vi "Ver 1.7.vi"() -> ()   [LabVIEW 2015]
uses:
  <instrlib>/Keithley 622x LV 2009/Configure/Source/Typedefs/KE622x -- Current Range.ctl
  <instrlib>/Keithley 622x LV 2009/Configure/Source/Typedefs/KE622x -- Current Ranges.ctl
  <instrlib>/Keithley 622x LV 2009/Typedefs/KE622x -- On Off Control.ctl
  <instrlib>/Keithley 622x LV 2009/Configure/Source/Typedefs/KE622x -- Voltage Limit.ctl
  <instrlib>/Keithley 622x LV 2009/Utility/Typedefs/KE622x -- Instrument Type.ctl
  <instrlib>/Keithley 2000/Public/Configure/Configure DC Volts.vi
  <userlib>/LV-Link3/PolySubVIs/DtCreateAinChan.vi
  <userlib>/LV-Link3/PolySubVIs/DtOLReadSingle.vi
  <instrlib>/Keithley 2000/Keithley 2000.lvlib
  <instrlib>/Keithley 622x LV 2009/Keithley 622x.lvlib
panel:
  out "MULTIPLE GRAPHS":cluster{dbl[], dbl[]}[](graph)
  in  "X-Axis":T1(ring)
  in  "Range":u8(ring)=20 items=["100nV", "200nV", "500nV", "1µV", "2µV", "5µV", "10µV", "20µV", "50µV", "100µV", "200µV", "500µV", "1mV", "2mV", "5mV", "10mV", "20mV", "50mV", "100mV", "200mV", "500mV", "1V"]
  in  "Display Type copy":u16(ring) items=["X %", "Y %", "X Calibrated", "Y Calibrated", "Mag %", "Mag Calibrated", "Phase Degrees", "Ratio", "ADC 1", "ADC 2", "ADC 3", "ADC 4 ", "Noise %", "Noise Calibrated", "Ref Frequency", "", ""]
  out "Units copy":string
  out "Display copy":dbl format="%.3f"
  out "Overload":bool
  out "Display":dbl format="%.3f"
  out "Units":string
  in  "Display Type":u16(ring) items=["X %", "Y %", "X Calibrated", "Y Calibrated", "Mag %", "Mag Calibrated", "Phase Degrees", "Ratio", "ADC 1", "ADC 2", "ADC 3", "ADC 4 ", "Noise %", "Noise Calibrated", "Ref Frequency", "", ""]
  in  "Time Constant":u16(ring) items=["MIN", "1ms", "3ms", "10ms", "30ms", "100ms", "300ms", "1s", "3s", "10s", "30s", "100s", "300s"]
  in  "Slope":u8(ring) items=["6db/octave", "12dB/octave"]
  in  "Dynamic Reserve":u16(ring) items=["High Stability", "Normal", "High Reserve"]
  in  "Auto Sensitivity":bool
  in  "Auto Measure":bool
  out "Task out":i32
  out "daq_error out":errorcluster
  out "6221_error_out":errorcluster
  out "2000_error_out":errorcluster
  out "5110_error_out":errorcluster
  out "Input Mode":i32(ring) items=[" Voltage Input (A or A-B) ", "Current Input 10E6 V/A", "Current Input 10E8 V/A"]
  out "5110":refnum<visa-resource-name>
  in  "GPIB Address":i8=12 min=1 max=32 step=1
  out "DAQ":dbl format="%#_13g"
  out "2000":dbl format="%#_13g"
  in  "Device":string(combo)
  in  "Channels":string="0"
  in  "Number \nof points":i32
  in  "Folder\nprename":string
  out "TIME GRAPH":cluster{dbl[], dbl[]}[](graph)
  out "T0":u32
  out "LIMIT":bool
  out "LIMIT":bool
  out "Error Code":string
  in  "Comments":string
  out "file":refnum<file>
  out "2000":refnum<visa-resource-name>
  out "6221":refnum<visa-resource-name>
  out "Step  (A)":dbl=5e-05 format="%#_3p"
  in  "Stop\ncurrent (A)":dbl=0.002 format="%#_6p"
  in  "Start \ncurrent (A)":dbl=0.001 format="%#_6p"
  in  "Check For SCPI Errors? (T)":bool=TRUE
  out "Interlock Tripped?":bool
  out "Compliance?":bool
  in  "Turn Off Output \nIf Compliance?":bool=TRUE
  in  "Turning ON/OFF\ncurrent output":T2=enum."On"
  in  "Range Selection":T3={"Auto Range?"=TRUE, "Man / Selected\nRange"=enum."2nA"}
  # "FILE CONFIGURATION"
  # "ADMIN PANEL"
  # "KEITHLEY 6221 CONFIGURATION (ADMIN ONLY)"
  # "KEITHLEY DAQ CONFIGURATION (ADMIN ONLY)"
  # "READINGS"
  # "PRINCETON LOCK-IN AMP (ADMIN ONLY)"
  # "I don't know what the hell it is,\njust don't touch it"
  # "SENSITIVITY"
  # "INPUT CONFIGURATION"
  # "START, STOP, STEP, CONFIGURATION"
  # "IF ON"
  # "Output Channels Time - Constant \nSlope & Dynamic Reserve"
  # "Compliance = Limiting output voltage\nThis switch determines if we want to switch \noff the current output if wee exceed compliance"
  # "LOCK-IN READINGS"
  # "RIGHT DISPLAY"
  # "LEFT DISPLAY"
  # "There is a safe switch at \nthe back of the instrument \nThis indicator shows if it is on"
  # "You have hit a damn jackpot \nby exceeding the limited voltage\nCongrats"
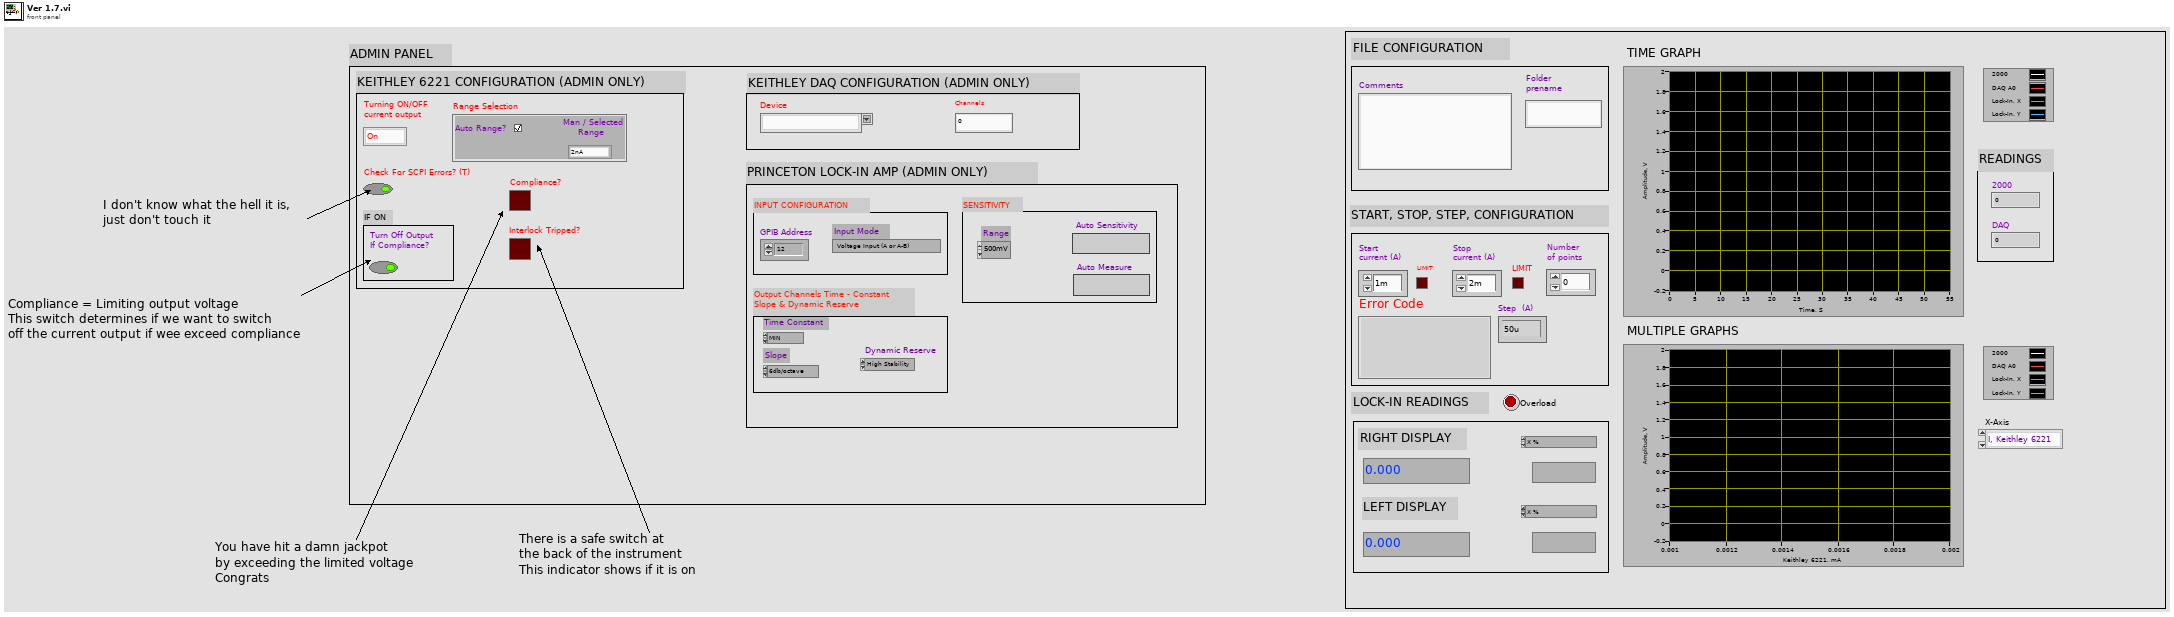
[diagram p1: front panel]
types:
  T1 = enum16{"I, Keithley 6221", "V, Keithley 2000", "V, Keithley DAQ", "V, Lock-In X", "V, Lock-In Y"}
  T2 = typedef "Keithley 622x.lvlib/KE622x -- On Off Control.ctl" = enum16{"Off", "On"}
  T3 = typedef "Keithley 622x.lvlib/KE622x -- Current Range.ctl" = cluster{"Auto Range?":bool, "Man / Selected\nRange":T4}
  T4 = typedef "Keithley 622x.lvlib/KE622x -- Current Ranges.ctl" = enum16{"2nA", "20nA", "200nA", "2uA", "20uA", "200uA", "2mA", "20mA", "100mA"}
  T5 = typedef "Keithley 622x.lvlib/KE622x -- Voltage Limit.ctl" = dbl
  T6 = typedef "Keithley 622x.lvlib/KE622x -- Instrument Type.ctl" = enum16{"KE6220", "KE6221"}
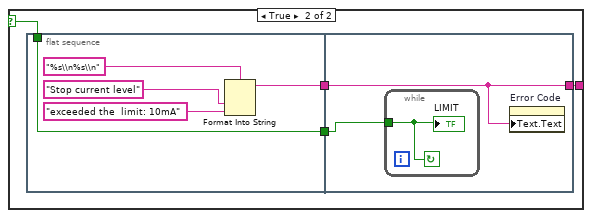
[diagram p2: hidden frame]
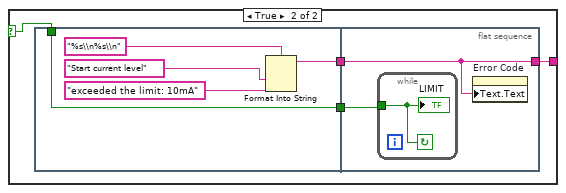
[diagram p3: hidden frame]
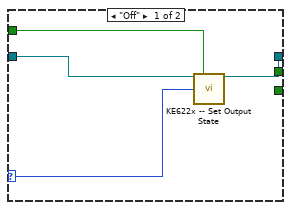
[diagram p4: hidden frame]
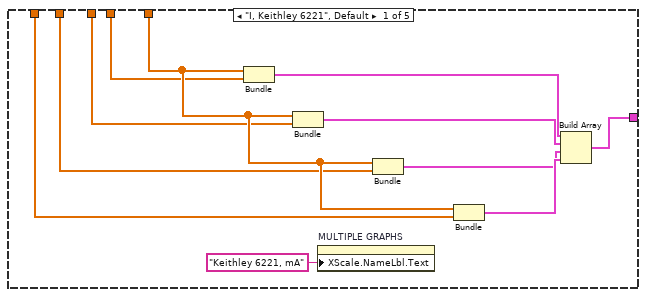
[diagram p5: hidden frame]
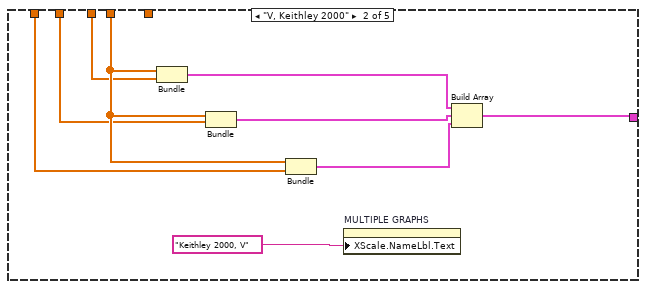
[diagram p6: hidden frame]
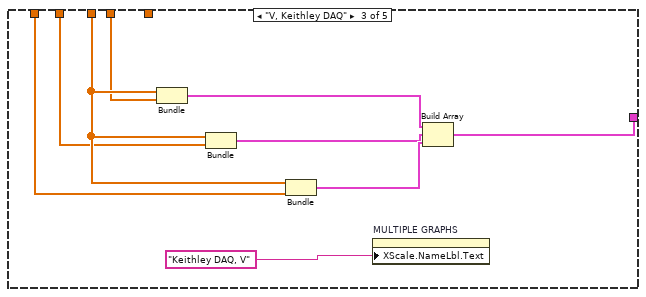
[diagram p7: hidden frame]
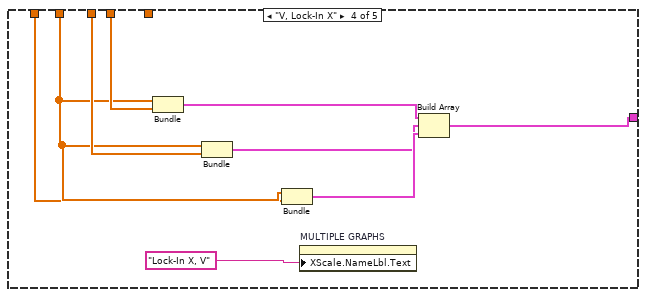
[diagram p8: hidden frame]
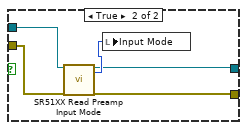
[diagram p9: hidden frame]
diagram:
  n1 = flat-sequence {
    tunnel: [w147] -> w8
    tunnel: [w145] -> w7
    tunnel: [w144] -> w6
    tunnel: [w143] -> w5
    tunnel: [w142] -> w4
    tunnel: [w141] -> w3
    tunnel: [w132] -> w2
    tunnel: [w131] -> w1
    tunnel: w8 -> [w543]
    tunnel: w7 -> [w542]
    tunnel: w6 -> [w541]
    tunnel: w5 -> [w540]
    tunnel: w4 -> [w539]
    tunnel: w3 -> [w538]
    tunnel: w2 -> [w537]
    tunnel: w1 -> [w536]
    frame #0 {
      # "Calculating steps by number\nof points"
      # "Time Intit"
      # "Putting in a loop \ninstead of \"STOP\""
      # "Start, Stop, Step"
      # "Initializing instruments"
      # "File configuration"
      n2 = flat-sequence {
        frame #0 {
          w31 = TRUE  # reset
          w30 = FALSE  # ID query
          # "Initialize Lock-In 5110"
          # "Initialize Keithley 2000"
          # "Initialize Keithley 6221"
          n3 = call <instrlib>:"Initialize.vi"("VISA resource name"=refnum<visa-resource-name> "KEITHLEY_MULTIMETER") -> ("VISA resource name out"=w35:refnum<visa-resource-name>)  [unwired: 17 in, 1 out]
          n4 = call <instrlib>:"Initialize.vi"("VISA resource name"=refnum<visa-resource-name> "KEITHLEY_DC_AC_CURRENT_SOURCE", "Error Queue Option"=enum16{"Clear Error Queue", "Error Query"}."Clear Error Queue", "Instrument Type"=KE622x_--_Instrument_Type."KE6221") -> ("VISA resource name out"=→"6221":refnum<visa-resource-name>, "error out"=→"6221_error_out":errorcluster)  [unwired: 11 in]
          n5 = call "SR51XX Initialize"("VISA session (for class)"=refnum<visa-resource-name> "LOCK_IN_5110_PRINCETON", "Interface"=FALSE, "ID query"=w30, "GPIB Address"="GPIB Address", "reset"=w31) -> ("VISA session"=→"5110":refnum<visa-resource-name>, "error out"=→"5110_error_out":errorcluster)  [unwired: 8 in, 1 out]
          n6 = call-poly <instrlib>:"Configure Measurement.vi"("VISA resource name"=w35) -> ("VISA resource name out"=→"2000":refnum<visa-resource-name>, "error out"=→"2000_error_out":errorcluster)  [unwired: 17 in]
        }
        frame #1 {
          # "Initialize Keithley DAQ \n(getting board name)"
          n7 = call <userlib>:"DtOLGetBoardNames.vi"() -> ("Number of boards"=w40:u32)  [unwired: 9 in, 2 out]
          n8 = Initialize Array("", w40) -> (w42:string[])
          n9 = for {
            N: w40 -> [_]
            shift-right: [w48] -> w45
            shift-left: w42 -> [w49]
            i -> [w47]
            n10 = Add(x=1, y=w47) -> (x+y=w51:i32)
            n11 = call <userlib>:"DtOLGetBoardNames.vi"("Select Board"=w51) -> ("Board Name"=w46:string)  [unwired: 8 in, 2 out]
            n12 = Replace Array Subset(array=w49, new element=w46, index=w47) -> (w48:string[])
          }
          n13 = Index Array(array=w45, index=0) -> (element=w44:string)
          n14 = property on="Device" class="CmbBox"("Strings[]"=w45, "Value"=w44) -> ()  [unwired: 2 in, 2 out]
        }
      }
      n15 = local read "Stop\ncurrent (A)"() -> (w12:dbl)
      n16 = local read "Start \ncurrent (A)"() -> (w11:dbl)
      n17 = Greater?(x="Start \ncurrent (A)", y=T5 0.01) -> (0:w19:bool)
      n18 = local write "Start \ncurrent (A)"("Start \ncurrent (A)") -> ()
      n19 = Subtract(x=w12, y=w11) -> (x-y=w9:dbl)
      n20 = Divide(x=w9, y="Number \nof points") -> (x/y=→"Step  (A)":dbl)
      n21 = Greater?(x="Stop\ncurrent (A)", y=T5 0.01) -> (0:w18:bool)
      n22 = local write "Stop\ncurrent (A)"("Stop\ncurrent (A)") -> ()
      n23 = case shown="False" w19 {
        selector: w19 -> [_ w71]
        tunnel: [w67 w73] -> w17
        frame False {
          n24 = Format Into String(format string="%s\\n", "Start current level is OK" ("false string")) -> (resulting string=w67:string)  [unwired: 2 in, 1 out]
        }
        frame True {
          n25 = flat-sequence {
            tunnel: [w75] -> w72
            tunnel: w71 -> [w74]
            tunnel: [w74] -> w70
            tunnel: [w79] -> w73
            tunnel: w72 -> [w79]
            tunnel: w70 -> [w80]
            frame #0 {
              n26 = Format Into String(format string="%s\\n%s\\n", "Start current level" ("String"), "exceeded the limit: 10mA" ("input 2")) -> (resulting string=w75:string)  [unwired: 2 in, 1 out]
            }
            frame #1 {
              n27 = while {
                tunnel: w80 -> [w81]
                stop <- w81 continue-if-true
                "LIMIT" <- w81
              }
              n28 = property on="Error Code" class="Str"("Text.Text"=w79) -> ()  [unwired: 2 in, 2 out]
            }
          }
        }
      }
      n29 = case shown="False" w18 {
        selector: w18 -> [_ w55]
        tunnel: [w52 w58] -> w16
        frame False {
          n30 = Format Into String(format string="%s\\n", "Start current level is OK" ("false string")) -> (resulting string=w52:string)  [unwired: 2 in, 1 out]
        }
        frame True {
          n31 = flat-sequence {
            tunnel: [w60] -> w57
            tunnel: [w59] -> w56
            tunnel: w55 -> [w59]
            tunnel: [w64] -> w58
            tunnel: w57 -> [w64]
            tunnel: w56 -> [w65]
            frame #0 {
              n32 = Format Into String(format string="%s\\n%s\\n", "Stop current level" ("String"), "exceeded the  limit: 10mA" ("input 2")) -> (resulting string=w60:string)  [unwired: 2 in, 1 out]
            }
            frame #1 {
              n33 = while {
                tunnel: w65 -> [w66]
                stop <- w66 continue-if-true
                "LIMIT" <- w66
              }
              n34 = property on="Error Code" class="Str"("Text.Text"=w64) -> ()  [unwired: 2 in, 2 out]
            }
          }
        }
      }
      n35 = flat-sequence {
        frame #0 {
          # "Creating folder&file"
          n36 = call "folder_creation.vi"("Name"="Folder\nprename") -> ("String"=w83:string)
          n37 = call "file_creation.vi"("String"=w83) -> ("refnum out"=→"file":refnum<file>)
        }
        frame #1 {
          # "Creating comments"
          n38 = local read "file"() -> (w85:refnum<file>)
          n39 = Format Into String(format string="#%s\\n", initial string=w85, "Comments") -> ()  [unwired: 1 in, 2 out]
        }
        frame #2 {
          # "Adding headlines"
          n40 = local read "file"() -> (w95:refnum<file>)
          n41 = Format Into String(format string="%s\\t%s\\t\\t%s\\t\\t%s\\t%s\\t\\t%s\\n", initial string=w95, "Sec" ("input 1"), "A" ("input 2"), "V" ("input 3"), "X " ("input 3"), "Y" ("input 3"), "Phase" ("input 3")) -> ()  [unwired: 1 in, 2 out]
        }
      }
      n42 = Concatenate Strings(w17, w16) -> (→"Error Code":string)
      n43 = Tick Count (ms)() -> (millisecond timer value=→"T0":u32)
    }
    frame #1 {
      # "Configuring Keithley DAQ just before measuments"
      # "Configuring Keithley 6221 just before measuments"
      n44 = flat-sequence {
        tunnel: [w106] -> w98
        tunnel: [w124] -> _
        tunnel: [w126] -> _
        tunnel: w98 -> [w125]
        frame #0 {
          # "Current range \nselection check"
          # "Checking for compliance\nand interlock errors"
          n45 = local read "6221"() -> (w109:refnum<visa-resource-name>)
          n46 = call <instrlib>:"KE622x -- Set Current Range.vi"("Resource In"=w109, "Current Range In"="Range Selection", "Read Back Set Values? (T)"=FALSE) -> ("Resource Out (dupl)"=w114:refnum<visa-resource-name>)  [unwired: 10 in, 2 out]
          n47 = case shown="\"On\"" "Turning ON/OFF\ncurrent output" {
            selector: "Turning ON/OFF\ncurrent output" -> [w118 _]
            tunnel: [_ w122] -> w112
            tunnel: [_ w121] -> w113
            tunnel: "Check For SCPI Errors? (T)" -> [w117 _]
            tunnel: w114 -> [w115 w120]
            tunnel: [w116 w119] -> w106
            frame "Off" {
              n48 = call <instrlib>:"KE622x -- Set Output State.vi"("Resource In"=w115, "Check For SCPI Errors? (T)"=w117, "Output State"=w118) -> ("Resource Out (dupl)"=w116:refnum<visa-resource-name>)  [unwired: 11 in, 1 out]
            }
            frame "On" {
              n49 = call <instrlib>:"KE622x -- Turn Output On And Check For Errors.vi"("Resource In"=w120, "Turn Off Output If Compliance?"="Turn Off Output \nIf Compliance?") -> ("Resource Out (dupl)"=w119:refnum<visa-resource-name>, "Interlock Tripped?"=w122:bool, "Compliance?"=w121:bool)  [unwired: 10 in, 1 out]
            }
          }
          "Interlock Tripped?" <- w112
          "Compliance?" <- w113
        }
        frame #1 {
          # "Setting start current"
          n50 = local read "Start \ncurrent (A)"() -> (w124:dbl)
          n51 = Wait (ms)(milliseconds to wait=u32 100) -> ()  [unwired: 1 out]
          n52 = call <instrlib>:"KE622x -- Set Current Level.vi"("Resource In"=w125, "Current Level (A) In"=w124) -> ("Resource Out (dupl)"=w126:refnum<visa-resource-name>)  [unwired: 12 in, 1 out]
        }
      }
      n53 = flat-sequence {
        tunnel: [w100] -> w96
        tunnel: [w99] -> w97
        frame #0 {
          w104 = 100 items=["SingleEnded"=100, "Differential"=101] ("Channel Type")
          # "Configure the input channel"
          n54 = call-poly <userlib>:"DtOLCreateTask.vi"("Channel Type"=w104, "Range Min"=-10.0, "Range Max"=10.0, "Board Name"="Device", "Channel"="Channels") -> ("Task out"=w100:i32, "error out"=w99:errorcluster)  [unwired: 8 in, 1 out]
        }
      }
      "daq_error out" <- w97
      "Task out" <- w96
    }
    frame #2 {
      # "Plotting the results"
      # "Creting plot from the DAQ data"
      # "Creting plot from the 2000 data"
      n55 = local read "5110_error_out"() -> (w137:errorcluster)
      n56 = local read "6221_error_out"() -> (w135:errorcluster)
      n57 = local read "2000_error_out"() -> (w133:errorcluster)
      n58 = local read "daq_error out"() -> (w136:errorcluster)
      n59 = local read "Task out"() -> (w134:i32)
      n60 = local read "5110"() -> (w138:refnum<visa-resource-name>)
      n61 = local read "2000"() -> (w140:refnum<visa-resource-name>)
      n62 = local read "6221"() -> (w139:refnum<visa-resource-name>)
      n63 = while {
        shift-right: [w154] -> _
        shift-left: dbl[] [] -> [w312]
        shift-right: [w170] -> _
        shift-left: i32[] [] -> [w311]
        tunnel: w140 -> [w309]
        tunnel: w139 -> [w308]
        tunnel: w136 -> [w295]
        tunnel: w134 -> [w291]
        tunnel: [w300] -> w147
        shift-right: [w153] -> _
        shift-left: dbl[] [] -> [w299]
        tunnel: [w286] -> w145
        tunnel: [w285] -> w144
        tunnel: [w284] -> w143
        tunnel: [w282] -> w142
        tunnel: [w279] -> w141
        tunnel: w138 -> [w271]
        tunnel: w137 -> [w268]
        tunnel: w135 -> [w258]
        tunnel: w133 -> [w256]
        tunnel: [w176] -> w132
        tunnel: [w173] -> w131
        shift-right: [w152] -> _
        shift-left: dbl[] [] -> [w172]
        shift-right: [w151] -> _
        shift-left: dbl[] [] -> [w171]
        shift-right: [w155] -> _
        shift-left: dbl[] [] -> [w157]
        i -> [w259]
        stop <- w301 stop-if-true
        # "Time"
        # "V, DAQ"
        # "V, 2000"
        n64 = Quotient & Remainder(x=w259, y=10) -> (floor(x/y)=w266:i32)  [unwired: 1 out]
        n65 = Equal?(x=0, y=w259) -> (x = y?=w263:bool)
        n66 = Equal?(x=1, y=w266) -> (x = y?=w261:bool)
        n67 = local read "T0"() -> (w310:u32)
        n68 = flat-sequence {
          tunnel: w309 -> [w371]
          tunnel: [w371] -> w275
          tunnel: w308 -> [w370]
          tunnel: [w370] -> w274
          tunnel: [w368] -> w273
          tunnel: w295 -> [w368]
          tunnel: [w367] -> w272
          tunnel: w291 -> [w367]
          tunnel: w271 -> [w366]
          tunnel: [w366] -> w270
          tunnel: [w365] -> w269
          tunnel: w268 -> [w365]
          tunnel: w263 -> [w364]
          tunnel: [w364] -> w262
          tunnel: w261 -> [w363]
          tunnel: [w363] -> w260
          tunnel: w258 -> [w362]
          tunnel: [w362] -> w257
          tunnel: w256 -> [w361]
          tunnel: [w361] -> w255
          tunnel: [w360] -> w246
          tunnel: w275 -> [w385]
          tunnel: [w385] -> w245
          tunnel: w274 -> [w384]
          tunnel: [w384] -> w244
          tunnel: w273 -> [w383]
          tunnel: [w383] -> w243
          tunnel: w272 -> [w382]
          tunnel: [w382] -> w242
          tunnel: w270 -> [w381]
          tunnel: w269 -> [w378]
          tunnel: [w377] -> w241
          tunnel: [w376] -> w240
          tunnel: w262 -> [w375]
          tunnel: [w375] -> w239
          tunnel: w260 -> [w374]
          tunnel: w257 -> [w373]
          tunnel: [w373] -> w238
          tunnel: w255 -> [w372]
          tunnel: [w372] -> w237
          tunnel: w245 -> [w411]
          tunnel: [w411] -> w236
          tunnel: w244 -> [w410]
          tunnel: [w410] -> w235
          tunnel: w243 -> [w409]
          tunnel: [w409] -> w234
          tunnel: w242 -> [w408]
          tunnel: [w408] -> w233
          tunnel: w241 -> [w405]
          tunnel: [w404] -> w232
          tunnel: w240 -> [w403]
          tunnel: [w402] -> w231
          tunnel: w239 -> [w400]
          tunnel: [w400] -> w230
          tunnel: w238 -> [w407]
          tunnel: [w407] -> w229
          tunnel: w237 -> [w406]
          tunnel: [w406] -> w228
          tunnel: ["Auto Measure"] -> w227
          tunnel: ["Auto Sensitivity"] -> w226
          tunnel: [w395] -> w225
          tunnel: w236 -> [w431]
          tunnel: [w431] -> w224
          tunnel: w235 -> [w430]
          tunnel: [w430] -> w223
          tunnel: w234 -> [w429]
          tunnel: [w429] -> w222
          tunnel: w233 -> [w428]
          tunnel: [w428] -> w221
          tunnel: w232 -> [w421]
          tunnel: w231 -> [w419]
          tunnel: [w418] -> w220
          tunnel: w230 -> [w425]
          tunnel: [w425] -> w219
          tunnel: w229 -> [w427]
          tunnel: [w427] -> w218
          tunnel: w228 -> [w426]
          tunnel: [w426] -> w217
          tunnel: w227 -> [w423]
          tunnel: [w423] -> w216
          tunnel: w226 -> [w424]
          tunnel: [w424] -> w215
          tunnel: w225 -> [w414]
          tunnel: [w414] -> w214
          tunnel: [w420] -> w213
          tunnel: ["Time Constant"] -> w212
          tunnel: ["Slope"] -> w211
          tunnel: w224 -> [w454]
          tunnel: [w454] -> w210
          tunnel: w223 -> [w453]
          tunnel: [w453] -> w209
          tunnel: w222 -> [w452]
          tunnel: [w452] -> w208
          tunnel: w221 -> [w451]
          tunnel: [w451] -> w207
          tunnel: w220 -> [w438]
          tunnel: [w437] -> w206
          tunnel: w219 -> [w450]
          tunnel: [w450] -> w205
          tunnel: w218 -> [w449]
          tunnel: [w449] -> w204
          tunnel: w217 -> [w448]
          tunnel: [w448] -> w203
          tunnel: w216 -> [w447]
          tunnel: [w447] -> w202
          tunnel: w215 -> [w446]
          tunnel: [w446] -> w201
          tunnel: w214 -> [w439]
          tunnel: [w439] -> w200
          tunnel: w213 -> [w443]
          tunnel: [w442] -> w199
          tunnel: w212 -> [w440]
          tunnel: [w440] -> w198
          tunnel: w211 -> [w445]
          tunnel: [w445] -> w197
          tunnel: [w432] -> w163
          tunnel: w210 -> [w477]
          tunnel: [w477] -> w196
          tunnel: w209 -> [w476]
          tunnel: [w476] -> w194
          tunnel: w208 -> [w475]
          tunnel: [w475] -> w192
          tunnel: w207 -> [w474]
          tunnel: [w474] -> w190
          tunnel: w206 -> [w460]
          tunnel: w205 -> [w473]
          tunnel: [w473] -> w188
          tunnel: w204 -> [w472]
          tunnel: [w472] -> w187
          tunnel: w203 -> [w471]
          tunnel: [w471] -> w185
          tunnel: w202 -> [w470]
          tunnel: [w470] -> w183
          tunnel: w201 -> [w469]
          tunnel: [w469] -> w182
          tunnel: w200 -> [w461]
          tunnel: w199 -> [w458]
          tunnel: [w457] -> w181
          tunnel: w198 -> [w462]
          tunnel: w197 -> [w463]
          tunnel: [w459] -> w179
          tunnel: [w456] -> w177
          tunnel: [w455] -> w160
          tunnel: w196 -> [w485]
          tunnel: [w485] -> w195
          tunnel: w194 -> [w484]
          tunnel: [w484] -> w193
          tunnel: w192 -> [w483]
          tunnel: [w483] -> w191
          tunnel: w190 -> [w482]
          tunnel: [w482] -> w189
          tunnel: w188 -> [_]
          tunnel: w187 -> [w481]
          tunnel: [w481] -> w186
          tunnel: w185 -> [w480]
          tunnel: [w480] -> w184
          tunnel: w183 -> [_]
          tunnel: w182 -> [_]
          tunnel: w181 -> [w479]
          tunnel: [w479] -> w180
          tunnel: w179 -> [w478]
          tunnel: [w478] -> w178
          tunnel: w177 -> [_]
          tunnel: [w488] -> w306
          tunnel: w195 -> [w488]
          tunnel: w193 -> [w496]
          tunnel: w259 -> [w498]
          tunnel: [w494] -> w301
          tunnel: [w486] -> w304
          tunnel: [w496] -> w303
          tunnel: [w493] -> w296
          tunnel: w191 -> [w493]
          tunnel: [w492] -> w292
          tunnel: w189 -> [w492]
          tunnel: w186 -> [w490]
          tunnel: w184 -> [w491]
          tunnel: [w491] -> w254
          tunnel: [w490] -> w253
          tunnel: [w489] -> w252
          tunnel: [w487] -> w251
          tunnel: w180 -> [w487]
          tunnel: w178 -> [w489]
          tunnel: [w486] -> w156
          tunnel: w306 -> [w511]
          tunnel: [w511] -> w305
          tunnel: w304 -> [w510]
          tunnel: w303 -> [w509]
          tunnel: [w508] -> w297
          tunnel: w296 -> [w508]
          tunnel: [w507] -> w293
          tunnel: w292 -> [w507]
          tunnel: [w506] -> w283
          tunnel: [w505] -> w280
          tunnel: w254 -> [w503]
          tunnel: w253 -> [w504]
          tunnel: w252 -> [w501]
          tunnel: w251 -> [w502]
          tunnel: [w503] -> w250
          tunnel: [w502] -> w247
          tunnel: [w501] -> w174
          tunnel: w305 -> [w520]
          tunnel: [w520] -> w307
          tunnel: [w518] -> w298
          tunnel: w297 -> [w518]
          tunnel: [w517] -> w294
          tunnel: w293 -> [w517]
          tunnel: w283 -> [w516]
          tunnel: [w516] -> w281
          tunnel: w280 -> [w515]
          tunnel: [w515] -> w278
          tunnel: w250 -> [w514]
          tunnel: [w514] -> w249
          tunnel: [w513] -> w248
          tunnel: w247 -> [w513]
          tunnel: [w512] -> w175
          tunnel: w174 -> [w512]
          tunnel: w307 -> [w535]
          tunnel: [w524] -> w302
          tunnel: [w533] -> w300
          tunnel: w298 -> [w532]
          tunnel: w294 -> [w531]
          tunnel: [w525] -> w290
          tunnel: [w530] -> w286
          tunnel: [w529] -> w285
          tunnel: [w528] -> w284
          tunnel: [w527] -> w282
          tunnel: w281 -> [w527]
          tunnel: [w526] -> w279
          tunnel: w278 -> [w526]
          tunnel: [w525] -> w277
          tunnel: [w524] -> w276
          tunnel: w249 -> [w523]
          tunnel: w248 -> [w522]
          tunnel: [w522] -> w176
          tunnel: w175 -> [w521]
          tunnel: [w521] -> w173
          frame #0 {
            # "Config delay"
            n69 = Wait Until Next ms Multiple(millisecond multiple=u32 500) -> (millisecond timer value=w360:u32)
          }
          frame #1 {
            n70 = case shown="False" w374 {
              tunnel: w381 -> [w387 w392]
              tunnel: [w386 w390] -> w380
              tunnel: [w387 w389] -> w379
              tunnel: w378 -> [w386 w388]
              frame False {
              }
              frame True {
                n71 = call "SR51XX Read Preamp Input Mode"("VISA session (for class)"=w392, "error in (no error)"=w388) -> ("VISA session"=w389:refnum<visa-resource-name>, "Input Mode"=w391:i32, "error out"=w390:errorcluster)  [unwired: 15 in]
                n72 = local write "Input Mode"(w391) -> ()
              }
            }
            n73 = call "SR51XX Configure Signal Channel Input"("VISA session (for class)"=w379, "error in (no error)"=w380, "Update"=w375) -> ("VISA session"=w377:refnum<visa-resource-name>, "error out"=w376:errorcluster)  [unwired: 15 in]
          }
          frame #2 {
            n74 = local read "Input Mode"() -> (w401:i32)
            n75 = call "SR51XX Configure Sensitivity"("VISA session (for class)"=w405, "Input Mode"=w401, "Range"="Range", "error in (no error)"=w403, "Auto Sensitivity"="Auto Sensitivity", "Auto Measure"="Auto Measure", "Update"=w400) -> ("Range Annotations Out[]"=w393:string[], "VISA session"=w404:refnum<visa-resource-name>, "Auto Sensitivity out"=w397:bool, "Auto Measure out"=w396:bool, "Range Out"=w395:u8, "error out"=w402:errorcluster)  [unwired: 7 in]
            n76 = local write "Auto Sensitivity"(w397) -> ()
            n77 = local write "Auto Measure"(w396) -> ()
            n78 = property on="Range" class="Ring (strict)"("Strings []"=w393) -> ()  [unwired: 2 in, 2 out]
            n79 = local write "Range"(w395) -> ()
          }
          frame #3 {
            n80 = Or(x=w424, y=w423) -> (x .or. y?=w422:bool)
            n81 = call "SR51XX Configure Output Channels - Slope, TC and Dyn Reserve"("VISA session (for class)"=w421, "Time Constant"="Time Constant", "Slope"="Slope", "Check TC"=w422, "Dynamic Reserve"="Dynamic Reserve", "error in (no error)"=w419, "Range"=w414, "Update"=w425) -> ("VISA session"=w420:refnum<visa-resource-name>, "Slope Out"=w415:u8, "Time Constant Out"=w416:u16, "error out"=w418:errorcluster)  [unwired: 8 in]
            n82 = local write "Slope"(w415) -> ()
            n83 = local write "Time Constant"(w416) -> ()
          }
          frame #4 {
            n84 = local read "Input Mode"() -> (w444:i32)
            n85 = call "SR5110 Read Output"("VISA session (for class)"=w443, "Input Mode"=w444, "Time Constant"=w440, "Display Type"="Display Type", "Range"=w439, "error in (no error)"=w438, "Slope"=w445) -> ("Units"=→"Units":string, "Display Precision"=w435:i32, "Display"=w432:dbl, "VISA session"=w442:refnum<visa-resource-name>, "Available Display Types Out"=w434:string[], "Overload"=→"Overload":bool, "error out"=w437:errorcluster)  [unwired: 4 in, 2 out]
            "Display" <- w432
            n86 = property on="Display" class="DigNum (strict)"("Precision"=w435) -> ()  [unwired: 2 in, 2 out]
            n87 = property on="Display Type" class="Ring (strict)"("Strings []"=w434) -> ()  [unwired: 2 in, 2 out]
          }
          frame #5 {
            n88 = local read "Input Mode"() -> (w468:i32)
            n89 = call "SR5110 Read Output"("VISA session (for class)"=w458, "Input Mode"=w468, "Time Constant"=w462, "Display Type"="Display Type copy", "Range"=w461, "error in (no error)"=w460, "Slope"=w463) -> ("Units"=→"Units copy":string, "Display Precision"=w464:i32, "Display"=w455:dbl, "VISA session"=w457:refnum<visa-resource-name>, "Reference Unlock"=w456:bool, "Available Display Types Out"=w465:string[], "error out"=w459:errorcluster)  [unwired: 4 in, 2 out]
            "Display copy" <- w455
            n90 = property on="Display copy" class="DigNum (strict)"("Precision"=w464) -> ()  [unwired: 2 in, 2 out]
            n91 = property on="Display Type copy" class="Ring (strict)"("Strings []"=w465) -> ()  [unwired: 2 in, 2 out]
          }
          frame #6 {
          }
          frame #7 {
            # "Changing input current"
            n92 = local read "Step  (A)"() -> (w499:dbl)
            n93 = local read "Start \ncurrent (A)"() -> (w500:dbl)
            n94 = Multiply(x=w499, y=w498) -> (x*y=w497:dbl)
            n95 = Add(x=w500, y=w497) -> (x+y=w486:dbl)
            n96 = local read "Stop\ncurrent (A)"() -> (w495:dbl)
            n97 = Greater Or Equal?(x=w486, y=w495) -> (x >= y?=w494:bool)
          }
          frame #8 {
            # "Setting 6221 current"
            n98 = call <instrlib>:"KE622x -- Set Current Level.vi"("Resource In"=w509, "Current Level (A) In"=w510, "error in (no error)"=w504) -> ("Resource Out (dupl)"=w505:refnum<visa-resource-name>, "error out"=w506:errorcluster)  [unwired: 11 in]
          }
          frame #9 {
            # "Delay before measuremens"
            n99 = Wait Until Next ms Multiple(millisecond multiple=u32 50) -> ()  [unwired: 1 out]
          }
          frame #10 {
            # "Getting the data from DAQ and 2000"
            n100 = call-poly <userlib>:"DtOLRead.vi"("error in (no error)"=w532, "Timeout"=1.0, "Task in"=w531) -> ("error out"=w528:errorcluster, "Data Out"=w525:dbl, "Task out"=w533:i32)  [unwired: 6 in]
            n101 = call <instrlib>:"Data Read Single.vi"("VISA resource name"=w535, "error in (no error)"=w523) -> ("VISA resource name out"=w529:refnum<visa-resource-name>, "Measurement"=w524:dbl, "error out"=w530:errorcluster)  [unwired: 13 in, 2 out]
          }
        }
        n102 = Subtract(x=w246, y=w310) -> (x-y=w167:u32)
        n103 = Divide(x=w167, y=u32 1000) -> (x/y=w165:dbl)
        n104 = Build Array (concatenate)(w157, w156) -> (w155:dbl[])
        n105 = Build Array (concatenate)(w311, w165) -> (w170:dbl[])
        n106 = Build Array (concatenate)(w312, w302) -> (w154:dbl[])
        n107 = Divide(x=w160, y=u32 1000) -> (x/y=w159:dbl)
        n108 = Divide(x=w163, y=u32 1000) -> (x/y=w162:dbl)
        n109 = Build Array (concatenate)(w299, w290) -> (w153:dbl[])
        n110 = Build Array (concatenate)(w172, w162) -> (w152:dbl[])
        n111 = Build Array (concatenate)(w171, w159) -> (w151:dbl[])
        n112 = Bundle(w170, w154) -> (w288:cluster{dbl[], dbl[]})  [unwired: 1 in]
        n113 = Bundle(w170, w153) -> (w287:cluster{dbl[], dbl[]})  [unwired: 1 in]
        n114 = Bundle(w170, w152) -> (w169:cluster{dbl[], dbl[]})  [unwired: 1 in]
        n115 = Bundle(w170, w151) -> (w168:cluster{dbl[], dbl[]})  [unwired: 1 in]
        n116 = Build Array(w288, w287, w169, w168) -> (→"TIME GRAPH":cluster{dbl[], dbl[]}[])
        n117 = case shown="\"V, Lock-In Y\"" "X-Axis" {
          tunnel: w155 -> [w319 _ _ _ _]
          tunnel: w154 -> [w318 w332 w340 w347 w358]
          tunnel: w153 -> [w317 w328 w341 w346 w357]
          tunnel: w152 -> [w316 w327 w339 w345 w356]
          tunnel: w151 -> [w315 w326 w338 w344 w359]
          tunnel: [w314 w325 w334 w343 w352] -> w150
          frame "I, Keithley 6221", Default {
            n118 = Bundle(w319, w318) -> (w320:cluster{dbl[], dbl[]})  [unwired: 1 in]
            n119 = Bundle(w319, w317) -> (w321:cluster{dbl[], dbl[]})  [unwired: 1 in]
            n120 = property on="MULTIPLE GRAPHS" class="XYGraph (strict)"("XScale.NameLbl.Text"="Keithley 6221, mA" ("X Scale.Name Label.Text")) -> ()  [unwired: 2 in, 2 out]
            n121 = Bundle(w319, w316) -> (w322:cluster{dbl[], dbl[]})  [unwired: 1 in]
            n122 = Bundle(w319, w315) -> (w323:cluster{dbl[], dbl[]})  [unwired: 1 in]
            n123 = Build Array(w320, w321, w322, w323) -> (w314:cluster{dbl[], dbl[]}[])
          }
          frame "V, Keithley 2000" {
            n124 = Bundle(w332, w328) -> (w331:cluster{dbl[], dbl[]})  [unwired: 1 in]
            n125 = Bundle(w332, w327) -> (w330:cluster{dbl[], dbl[]})  [unwired: 1 in]
            n126 = Bundle(w332, w326) -> (w329:cluster{dbl[], dbl[]})  [unwired: 1 in]
            n127 = property on="MULTIPLE GRAPHS" class="XYGraph (strict)"("XScale.NameLbl.Text"="Keithley 2000, V" ("X Scale.Name Label.Text")) -> ()  [unwired: 2 in, 2 out]
            n128 = Build Array(w331, w330, w329) -> (w325:cluster{dbl[], dbl[]}[])
          }
          frame "V, Keithley DAQ" {
            n129 = Bundle(w341, w340) -> (w335:cluster{dbl[], dbl[]})  [unwired: 1 in]
            n130 = Bundle(w341, w339) -> (w336:cluster{dbl[], dbl[]})  [unwired: 1 in]
            n131 = Bundle(w341, w338) -> (w337:cluster{dbl[], dbl[]})  [unwired: 1 in]
            n132 = property on="MULTIPLE GRAPHS" class="XYGraph (strict)"("XScale.NameLbl.Text"="Keithley DAQ, V" ("X Scale.Name Label.Text")) -> ()  [unwired: 2 in, 2 out]
            n133 = Build Array(w335, w336, w337) -> (w334:cluster{dbl[], dbl[]}[])
          }
          frame "V, Lock-In X" {
            n134 = Bundle(w345, w347) -> (w348:cluster{dbl[], dbl[]})  [unwired: 1 in]
            n135 = Bundle(w345, w346) -> (w349:cluster{dbl[], dbl[]})  [unwired: 1 in]
            n136 = Bundle(w345, w344) -> (w350:cluster{dbl[], dbl[]})  [unwired: 1 in]
            n137 = property on="MULTIPLE GRAPHS" class="XYGraph (strict)"("XScale.NameLbl.Text"="Lock-In X, V" ("X Scale.Name Label.Text")) -> ()  [unwired: 2 in, 2 out]
            n138 = Build Array(w348, w349, w350) -> (w343:cluster{dbl[], dbl[]}[])
          }
          frame "V, Lock-In Y" {
            n139 = Bundle(w358, w359) -> (w355:cluster{dbl[], dbl[]})  [unwired: 1 in]
            n140 = Bundle(w357, w359) -> (w354:cluster{dbl[], dbl[]})  [unwired: 1 in]
            n141 = Bundle(w356, w359) -> (w353:cluster{dbl[], dbl[]})  [unwired: 1 in]
            n142 = property on="MULTIPLE GRAPHS" class="XYGraph (strict)"("XScale.NameLbl.Text"="Lock-In Y, V" ("X Scale.Name Label.Text")) -> ()  [unwired: 2 in, 2 out]
            n143 = Build Array(w355, w354, w353) -> (w352:cluster{dbl[], dbl[]}[])
          }
        }
        "MULTIPLE GRAPHS" <- w150
        "2000" <- w276
        "DAQ" <- w277
      }
    }
    frame #3 {
      # "Closing instrumental \nconnections"
      n144 = call <instrlib>:"Close.vi"("VISA resource name"=w541, "error in (no error)"=w542) -> ()  [unwired: 17 in, 1 out]
      n145 = call <userlib>:"DtOLCloseTask.vi"("Error in"=w540, "Task in"=w543) -> ("Error Out"=w544:errorcluster)  [unwired: 9 in]
      n146 = call <instrlib>:"Close.vi"("VISA resource name"=w538, "error in (no error)"=w539) -> ()  [unwired: 13 in, 1 out]
      n147 = call "SR51XX Close"("error in (no error)"=w536, "VISA session"=w537) -> ()  [unwired: 1 out]
      n148 = call <vilib>:"Simple Error Handler.vi"("error in (no error)"=w544) -> ()  [unwired: 4 in, 5 out]
    }
  }
